vi "Get Number of Links.vi"(8 "error in (no error)":errorcluster, 11 "Robot Arm in":refnum<class "Robot Arm.lvclass">) -> (0 "error out":errorcluster, 2 "number of links":i32, 3 "Robot Arm out":refnum<class "Robot Arm.lvclass">)   [LabVIEW 2013, in "Robot Arm.lvclass"]
uses:
  Robot Arm.lvclass
  Robot Arm.lvclass/Robot Arm.ctl
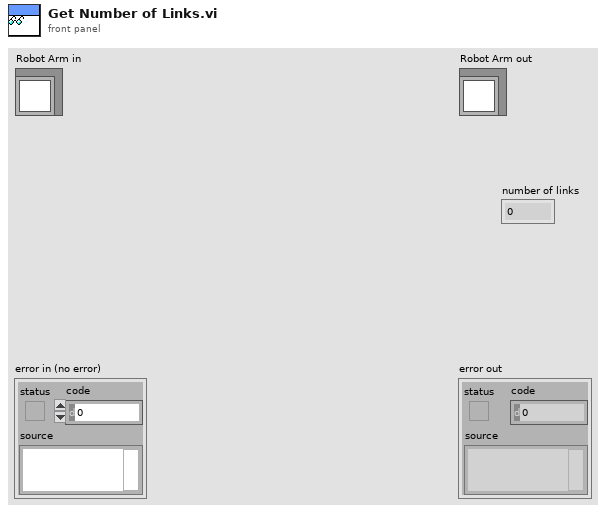
[diagram p1: front panel]
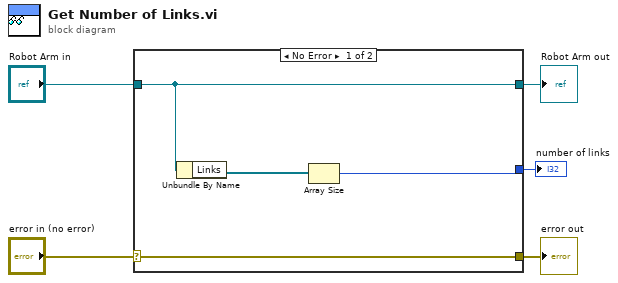
[diagram p0: block diagram]
diagram:
  n1 = case shown="No Error" "error in (no error)" {
    selector: "error in (no error)" -> [w9 w10]
    tunnel: [w9 w10] -> w4
    tunnel: [w8 w11] -> w2
    tunnel: "Robot Arm in" -> [w8 w11]
    tunnel: [w6 _] -> w1
    frame No Error {
      n2 = Unbundle By Name(w8) -> ("Links"=w7:refnum<class "Link.lvclass">[])
      n3 = Array Size(array=w7) -> (size(s)=w6:i32)
    }
    frame Error {
    }
  }
  "error out" <- w4
  "Robot Arm out" <- w2
  "number of links" <- w1
